vi "New PS Control Check (RT).vi"() -> ()   [LabVIEW 2019]
panel:
  out "Array 4":errorcluster[](array[cluster])
  out "Array 3":errorcluster[](array[cluster])
  in  "Array 2":bool[](array[boolean])
  in  "Array":dbl[](array[numeric])
  in  "stop":bool
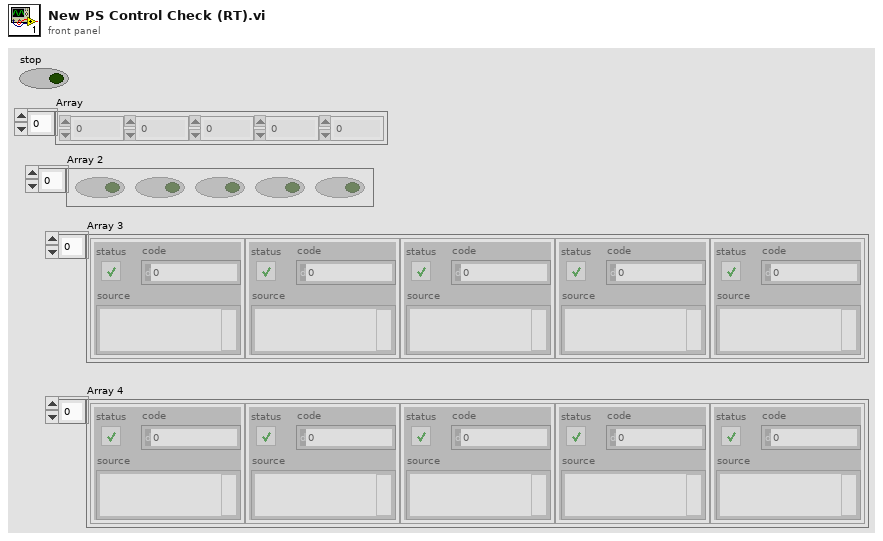
[diagram p1: front panel]
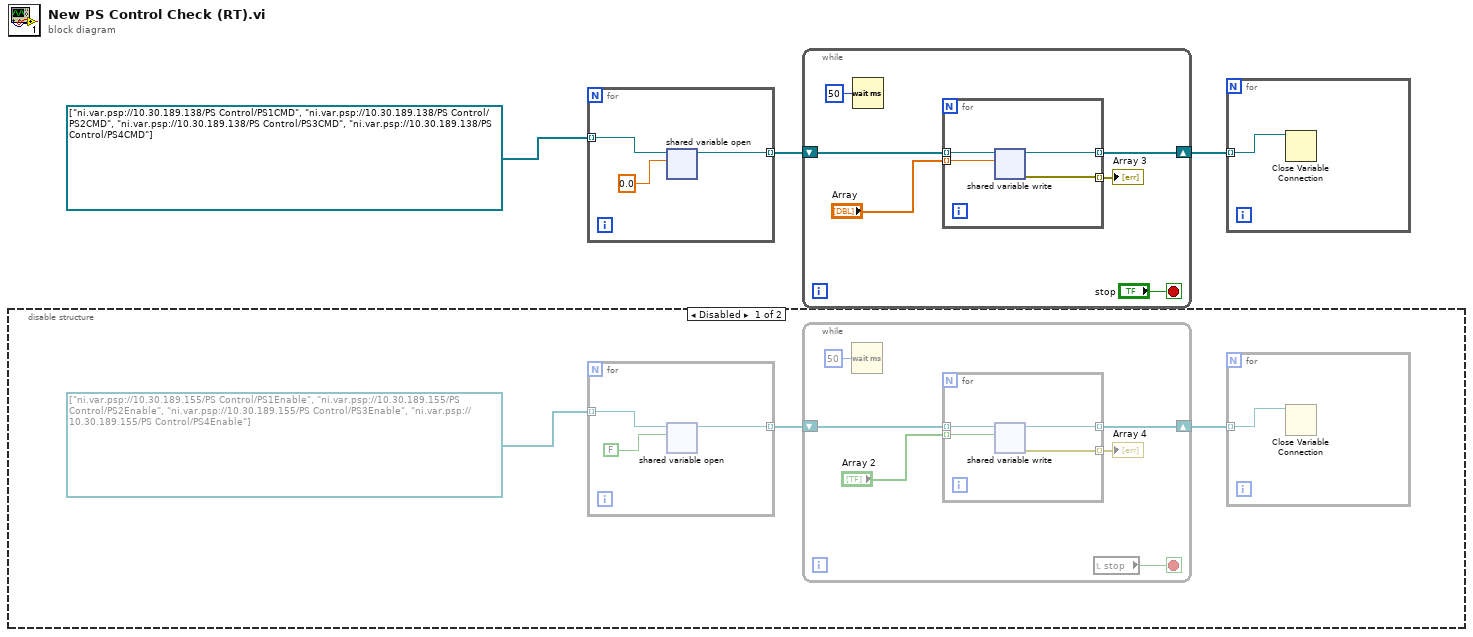
[diagram p0: block diagram]
diagram:
  n1 = disable-structure shown="Disabled" {
    frame Disabled {
      n2 = for {
        tunnel: refnum<k21>[] ["ni.var.psp://10.30.189.155/PS Control/PS1Enable", "ni.var.psp://10.30.189.155/PS Control/PS2Enable", "ni.var.psp://10.30.189.155/PS Control/PS3Enable", "ni.var.psp://10.30.189.155/PS Control/PS4Enable"] -> [w10] mode=indexing
        tunnel: [w9] -> w5 mode=indexing
        n3 = shared-variable-open(w10, FALSE) -> (w9:refnum<k21>)  [unwired: 2 in, 1 out]
      }
      n4 = while {
        shift-right: [w15] -> w6
        shift-left: w5 -> [w16]
        stop <- w13 stop-if-true
        n5 = Wait (ms)(milliseconds to wait=u32 50) -> ()  [unwired: 1 out]
        n6 = for {
          tunnel: w16 -> [w20] mode=indexing
          tunnel: [w19] -> w15 mode=indexing
          tunnel: "Array 2" -> [w18] mode=indexing
          tunnel: [w17] -> w11 mode=indexing
          n7 = shared-variable-write(w20, w18) -> (w19:refnum<k21>, w17:errorcluster)  [unwired: 1 in]
        }
        "Array 4" <- w11
        n8 = local read "stop"() -> (w13:bool)
      }
      n9 = for {
        tunnel: w6 -> [w7] mode=indexing
        n10 = Close Variable Connection(11:w7) -> ()  [unwired: 1 in, 1 out]
      }
    }
    frame Enabled {
    }
  }
  n11 = for {
    tunnel: refnum<k21>[] ["ni.var.psp://10.30.189.138/PS Control/PS1CMD", "ni.var.psp://10.30.189.138/PS Control/PS2CMD", "ni.var.psp://10.30.189.138/PS Control/PS3CMD", "ni.var.psp://10.30.189.138/PS Control/PS4CMD"] -> [w22] mode=indexing
    tunnel: [w21] -> w2 mode=indexing
    n12 = shared-variable-open(w22, 0.0) -> (w21:refnum<k21>)  [unwired: 2 in, 1 out]
  }
  n13 = while {
    shift-right: [w28] -> w1
    shift-left: w2 -> [w29]
    stop <- "stop" stop-if-true
    n14 = Wait (ms)(milliseconds to wait=u32 50) -> ()  [unwired: 1 out]
    n15 = for {
      tunnel: w29 -> [w33] mode=indexing
      tunnel: [w32] -> w28 mode=indexing
      tunnel: "Array" -> [w31] mode=indexing
      tunnel: [w30] -> w24 mode=indexing
      n16 = shared-variable-write(w33, w31) -> (w32:refnum<k21>, w30:errorcluster)  [unwired: 1 in]
    }
    "Array 3" <- w24
  }
  n17 = for {
    tunnel: w1 -> [w34] mode=indexing
    n18 = Close Variable Connection(11:w34) -> ()  [unwired: 1 in, 1 out]
  }
